vi "Ball Align(SubVI).vi"(0 "Align X - t, Y - f":bool, 2 "accuracy":u32=100, 3 "x is in range":bool, 4 "y is in range":bool, 5 "L_PWM":dbl=0.3, 6 "R_PWM":dbl=0.3, 7 "curX":dbl, 8 "defY":dbl, 9 "curY":dbl, 14 "defX":dbl, 16 "RangeY":dbl, 18 "RangeX":dbl) -> (13 "x_is_in_range":bool, 15 "y_is_in_range":bool, 20 "Align_X-t,Y-f":bool, 21 "Boolean 4":bool, 22 "accuracy out":u32=100, 23 "Boolean":bool, 24 "Boolean 3":bool, 25 "Boolean 2":bool, 26 "L_PWM out":dbl, 27 "R_PWM out":dbl)   [LabVIEW 2017]
panel:
  out "DEF R_PWM":dbl
  out "DEF L_PWM":dbl
  in  "extra power":dbl=0.2 format="%#_13g"
  in  "range for boost":dbl=250.0
  out "offset":bool
  in  "M_offsetX":dbl=30.0
  in  "M_defY":dbl=250.0
  # "IN"
  # "OUT"
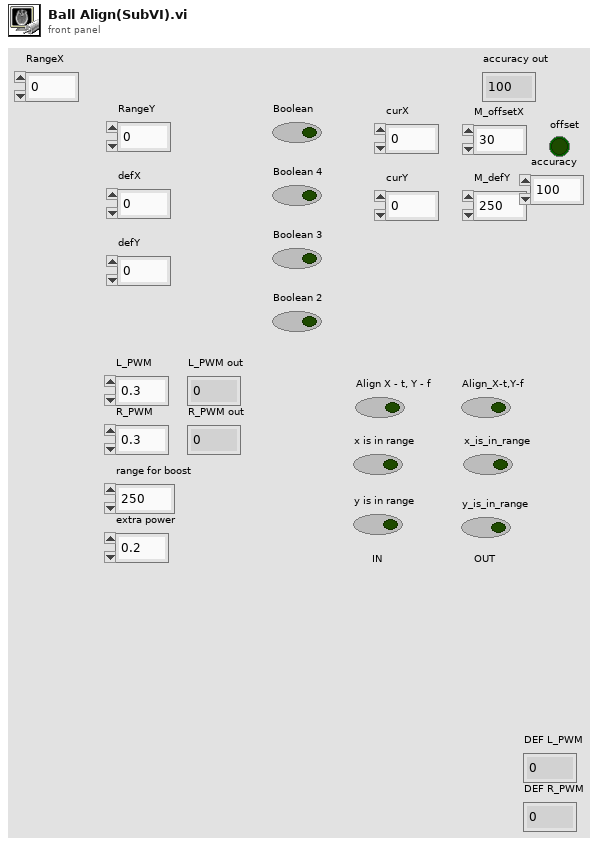
[diagram p1: front panel]
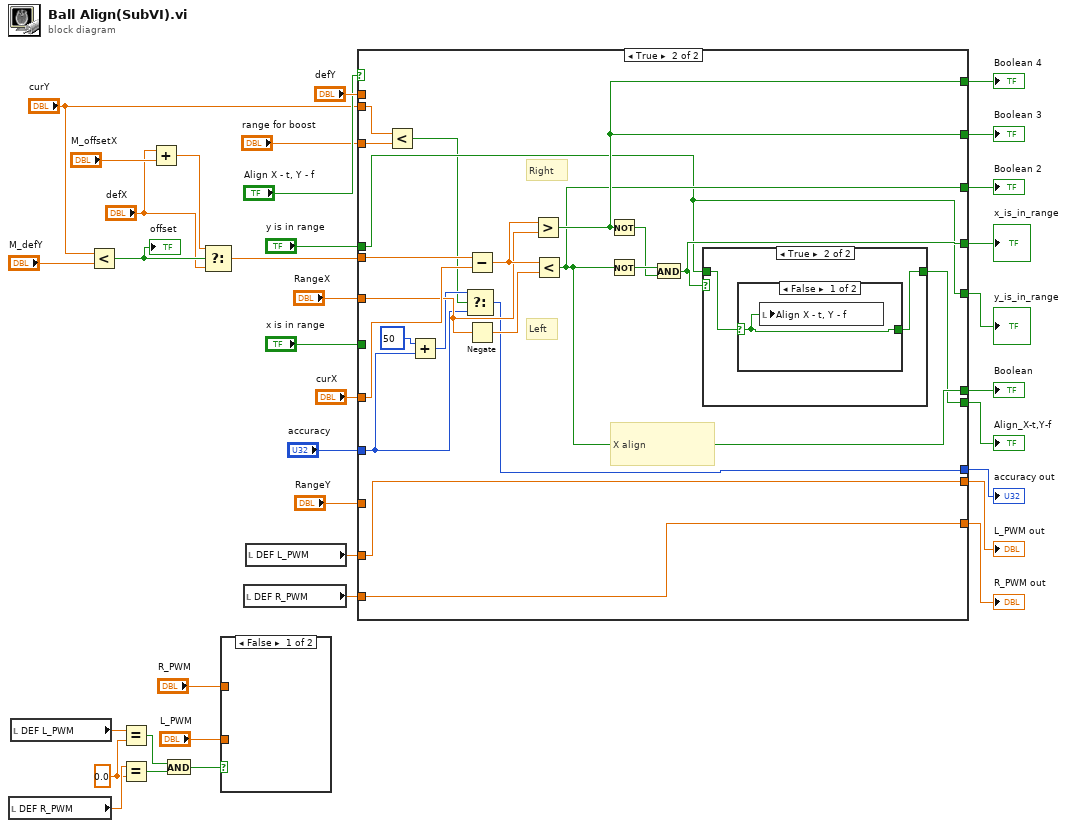
[diagram p0: block diagram]
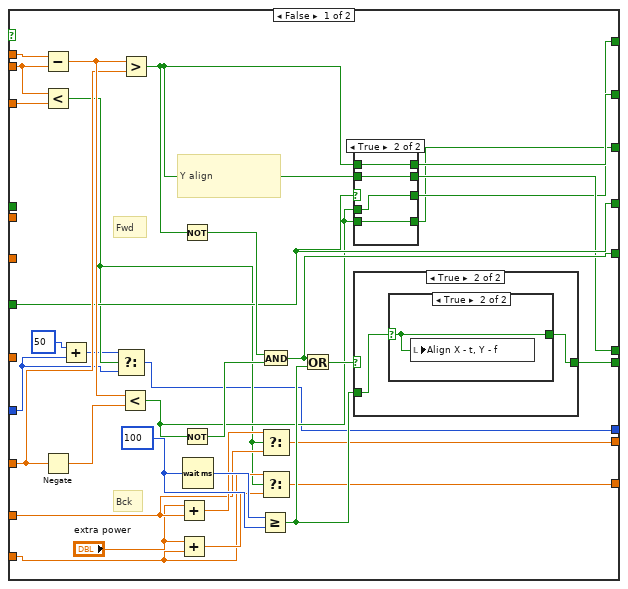
[diagram p2: hidden frame]
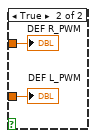
[diagram p8: hidden frame]
diagram:
  w10 = 0.0 ("y")
  n1 = local read "DEF R_PWM"() -> (w11:dbl)
  n2 = local read "DEF L_PWM"() -> (w12:dbl)
  n3 = Less?(x="curY", y="M_defY") -> (x < y?=w25:bool)
  "offset" <- w25
  n4 = Equal?(x=w12, y=w10) -> (x = y?=w8:bool)
  n5 = Equal?(x=w11, y=w10) -> (x = y?=w7:bool)
  n6 = Add(x="defX", y="M_offsetX") -> (x+y=w23:dbl)
  n7 = And(x=w8, y=w7) -> (x .and. y?=w9:bool)
  n8 = Select(t=w23, s=w25, f="defX") -> (s? t:f=w21:dbl)
  n9 = case shown="False" w9 {
    tunnel: "L_PWM" -> [_ w38]
    tunnel: "R_PWM" -> [_ w37]
    frame False {
    }
    frame True {
      "DEF L_PWM" <- w38
      "DEF R_PWM" <- w37
    }
  }
  n10 = local read "DEF R_PWM"() -> (w6:dbl)
  n11 = local read "DEF L_PWM"() -> (w5:dbl)
  n12 = case shown="True" "Align X - t, Y - f" {
    tunnel: w21 -> [_ w98]
    tunnel: "curX" -> [_ w97]
    tunnel: "RangeY" -> [w68 _]
    tunnel: "defY" -> [w69 _]
    tunnel: "curY" -> [w59 w85]
    tunnel: [w67 w93] -> w31
    tunnel: [w51 w96] -> w32
    tunnel: [w48 w95] -> w33
    tunnel: [w49 w95] -> w34
    tunnel: [w47 w94] -> w35
    tunnel: [w50 w94] -> w36
    tunnel: "x is in range" -> [w51 _]
    tunnel: "y is in range" -> [_ w93]
    tunnel: [w60 w92] -> w17
    tunnel: w5 -> [w57 w90]
    tunnel: w6 -> [w54 w91]
    tunnel: [w53 w90] -> w16
    tunnel: [w52 w91] -> w15
    tunnel: "RangeX" -> [_ w89]
    tunnel: "accuracy" -> [w44 w83]
    tunnel: [w40 w82] -> w2
    tunnel: "range for boost" -> [w39 w86]
    frame False {
      w63 = u32 100 ("milliseconds to wait")
      # "Bck"
      # "Fwd"
      # "Y align"
      n13 = Subtract(x=w69, y=w59) -> (x-y=w71:dbl)
      n14 = Less?(x=w59, y=w39) -> (x < y?=w43:bool)
      n15 = Negate(x=w68) -> (-x=w70:dbl)
      n16 = Add(x=u32 50, y=w44) -> (x+y=w42:u32)
      n17 = Select(t=w42, s=w43, f=w44) -> (s? t:f=w40:u32)
      n18 = Less?(x=w71, y=w70) -> (x < y?=w45:bool)
      n19 = Greater?(x=w71, y=w68) -> (0:w46:bool)
      n20 = Add(x="extra power", y=w57) -> (x+y=w58:dbl)
      n21 = Add(x="extra power", y=w54) -> (x+y=w56:dbl)
      n22 = Not(x=w46) -> (.not. x?=w66:bool)
      n23 = Not(x=w45) -> (.not. x?=w65:bool)
      n24 = Wait (ms)(milliseconds to wait=w63) -> (millisecond timer value=w64:u32)
      n25 = Greater Or Equal?(x=w64, y=w63) -> (x >= y?=w61:bool)
      n26 = And(x=w66, y=w65) -> (x .and. y?=w67:bool)
      n27 = Select(t=w58, s=w43, f=w57) -> (s? t:f=w53:dbl)
      n28 = Select(t=w54, s=w43, f=w56) -> (s? t:f=w52:dbl)
      n29 = Or(x=w67, y=w61) -> (x .or. y?=w62:bool)
      n30 = case shown="True" w51 {
        selector: w51 -> [w72 _]
        tunnel: [w72 w76] -> w50
        tunnel: w46 -> [_ w76]
        tunnel: w46 -> [_ w75]
        tunnel: [w72 w75] -> w49
        tunnel: w45 -> [_ w74]
        tunnel: [w72 w74] -> w48
        tunnel: w45 -> [_ w73]
        tunnel: [w72 w73] -> w47
        frame False {
        }
        frame True {
        }
      }
      n31 = case shown="True" w62 {
        selector: w62 -> [w77 _]
        tunnel: w61 -> [_ w79]
        tunnel: [w77 w78] -> w60
        frame False {
        }
        frame True {
          n32 = case shown="True" w79 {
            selector: w79 -> [w80 w81]
            tunnel: [w80 w81] -> w78
            frame False {
            }
            frame True {
              n33 = local write "Align X - t, Y - f"(w81) -> ()
            }
          }
        }
      }
    }
    frame True {
      # "X align"
      # "Right"
      # "Left"
      n34 = Less?(x=w85, y=w86) -> (x < y?=w84:bool)
      n35 = Add(x=u32 50, y=w83) -> (x+y=w88:u32)
      n36 = Select(t=w88, s=w84, f=w83) -> (s? t:f=w82:u32)
      n37 = Subtract(x=w98, y=w97) -> (x-y=w102:dbl)
      n38 = Negate(x=w89) -> (-x=w101:dbl)
      n39 = Greater?(x=w102, y=w89) -> (0:w95:bool)
      n40 = Less?(x=w102, y=w101) -> (x < y?=w94:bool)
      n41 = Not(x=w95) -> (.not. x?=w99:bool)
      n42 = Not(x=w94) -> (.not. x?=w100:bool)
      n43 = And(x=w100, y=w99) -> (x .and. y?=w96:bool)
      n44 = case shown="True" w96 {
        tunnel: w93 -> [w103 w105]
        tunnel: [w103 w104] -> w92
        frame False {
        }
        frame True {
          n45 = case shown="False" w105 {
            selector: w105 -> [w106 w107]
            tunnel: [w106 w107] -> w104
            frame False {
              n46 = local write "Align X - t, Y - f"(w106) -> ()
            }
            frame True {
            }
          }
        }
      }
    }
  }
  "Boolean" <- w36
  "Boolean 2" <- w35
  "Boolean 3" <- w34
  "Boolean 4" <- w33
  "x_is_in_range" <- w32
  "y_is_in_range" <- w31
  "Align_X-t,Y-f" <- w17
  "L_PWM out" <- w16
  "R_PWM out" <- w15
  "accuracy out" <- w2
